vi "ChangeParentClass.vi"(8 "error in (no error)":errorcluster, 10 "NewParentClass":string, 11 "CS++Actor in":refnum<class "CS++Actor.lvclass">) -> (0 "error out":errorcluster, 2 "Found?":bool, 3 "CS++Actor out":refnum<class "CS++Actor.lvclass">)   [LabVIEW 2014, in "CS++Actor.lvlib" / "CS++Actor.lvclass"]
doc: "Changes the inheritance of a class.\n\n<b>Note:</b> The new class has to be included in the target project."
uses:
  CS++Actor.lvclass
  CS++Actor.lvclass/CS++Actor.ctl
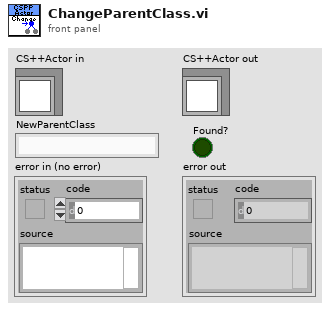
[diagram p1: front panel]
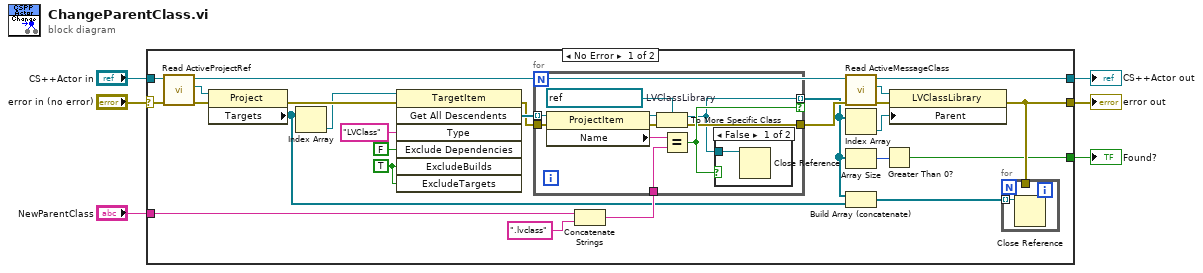
[diagram p0: block diagram]
diagram:
  n1 = case shown="No Error" "error in (no error)" {
    selector: "error in (no error)" -> [w17 w46]
    tunnel: [w12 w46] -> w5
    tunnel: [w32 w45] -> w3
    tunnel: "CS++Actor in" -> [w16 w45]
    tunnel: [w8 _] -> w2
    tunnel: "NewParentClass" -> [w7 _]
    frame No Error {
      w24 = TRUE ("ExcludeDependencies")
      n2 = call "Read ActiveProjectRef.vi"("error in (no error)"=w17, "CS++Actor in"=w16) -> ("error out"=w19:errorcluster, "ActiveProjectRef"=w18:refnum<vi>, "CS++Actor out"=w15:refnum<class "CS++Actor.lvclass">)  [unwired: 7 in]
      n3 = property class="Project"(reference=w18, error in=w19) -> (error out=w26:errorcluster, "Targets"=w22:refnum<vi>[])  [unwired: 1 out]
      n4 = Index Array(array=w22) -> (element=w20:refnum<vi>)  [unwired: 1 in]
      n5 = invoke class="TargetItem" method="Get All Descendents"(reference=w20, error in=w26, "Type"="LVClass", "Exclude Dependencies"=FALSE ("ExcludeDependencies"), "ExcludeBuilds"=w24, "ExcludeTargets"=w24) -> (error out=w21:errorcluster, "All Descendents"=w25:refnum<vi>[])  [unwired: 1 in, 5 out]
      n6 = Concatenate Strings(w7, ".lvclass" ("regular expression")) -> (w29:string)
      n7 = for {
        tunnel: w25 -> [w43] mode=indexing
        tunnel: w29 -> [w41]
        tunnel: [w35] -> w10 mode=indexing if=w39
        tunnel: w21 -> [w40]
        tunnel: [w37] -> w14
        w34 = refnum<vi> refnum  # LVClassLibrary
        n8 = property class="ProjectItem"(reference=w43, error in=w40) -> (reference out=w36:refnum<vi>, error out=w38:errorcluster, "Name"=w42:string)
        n9 = To More Specific Class(target class=w34, reference=w36, error in=w38) -> (specific class reference=w35:refnum<vi>, error out=w37:errorcluster)
        n10 = Equal?(x=w42, y=w41) -> (x = y?=w39:bool)
        n11 = case shown="False" w39 {
          tunnel: w35 -> [w44 _]
          frame False {
            n12 = Close Reference(reference=w44) -> ()  [unwired: 1 in, 1 out]
          }
          frame True {
          }
        }
      }
      n13 = call "Read ActiveMessageClass.vi"("error in (no error)"=w14, "CS++Actor in"=w15) -> ("error out"=w30:errorcluster, "ActiveMessageClass"=w31:refnum<vi>, "CS++Actor out"=w32:refnum<class "CS++Actor.lvclass">)  [unwired: 7 in]
      n14 = Index Array(array=w10) -> (element=w13:refnum<vi>)  [unwired: 1 in]
      n15 = Array Size(array=w10) -> (size(s)=w9:i32)
      n16 = Build Array (concatenate)(w10, w22) -> (w11:refnum<vi>[])
      n17 = Greater Than 0?(x=w9) -> (x > 0?=w8:bool)
      n18 = property class="LVClassLibrary"(reference=w31, error in=w30, "Parent"=w13) -> (error out=w12:errorcluster)  [unwired: 1 out]
      n19 = for {
        tunnel: w11 -> [w33] mode=indexing
        tunnel: w12 -> [_]
        n20 = Close Reference(reference=w33) -> ()  [unwired: 1 in, 1 out]
      }
    }
    frame Error {
    }
  }
  "error out" <- w5
  "CS++Actor out" <- w3
  "Found?" <- w2
